vi "create_or_update_indexFile.vi"(1 "html code":string, 2 "folder name":string) -> (0 "status":string)   [LabVIEW 2014]
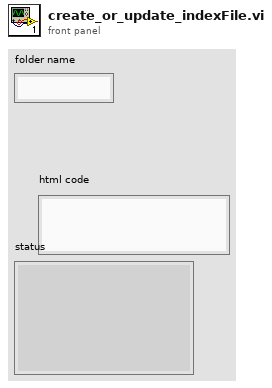
[diagram p1: front panel]
types:
  T1 = enum16{"open", "replace", "create", "open or create", "replace or create", "replace or create with confirmation"}
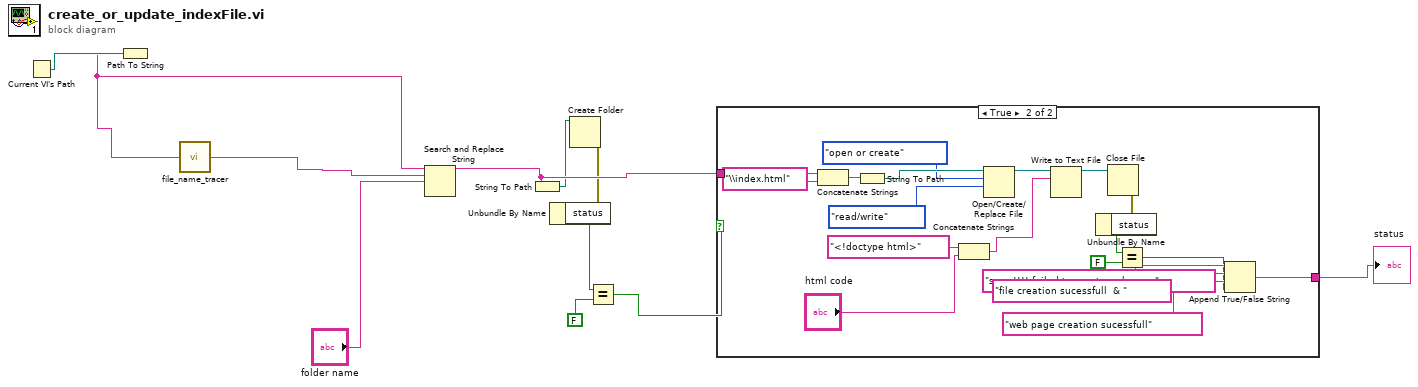
[diagram p0: block diagram]
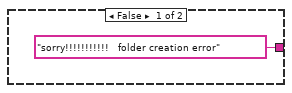
[diagram p2: hidden frame]
diagram:
  n1 = Current VI's Path() -> (path=w8:path)
  n2 = Path To String(path=w8) -> (string=w2:string)
  n3 = call "file_name_tracer.vi"("input path string"=w2) -> ("file name"=w1:string)
  n4 = Search and Replace String(input string=w2, search string=w1, replace string="folder name") -> (result string=w9:string)  [unwired: 5 in, 3 out]
  n5 = String To Path(string=w9) -> (path=w7:path)
  n6 = Create Folder(path (use dialog)=w7) -> (error out=w6:errorcluster)  [unwired: 2 in, 2 out]
  n7 = Unbundle By Name(w6) -> ("status"=w5:bool)
  n8 = Equal?(x=w5, y=FALSE) -> (x = y?=w11:bool)
  n9 = case shown="True" w11 {
    tunnel: ["sorry!!!!!!!!!!!   folder creation error" ("output string") w14] -> w10
    tunnel: w9 -> [_ w13]
    frame False {
    }
    frame True {
      n10 = Concatenate Strings(w13, "\\index.html" ("string")) -> (w30:string)
      n11 = String To Path(string=w30) -> (path=w29:path)
      n12 = Concatenate Strings("<!doctype html>" ("string"), "html code") -> (w23:string)
      n13 = Open/Create/Replace File(file path (use dialog)=w29, operation (0:open)=T1."open or create", access (0:read/write)=enum16{"read/write", "read-only", "write-only"}."read/write") -> (refnum out=w26:refnum<file>)  [unwired: 3 in, 2 out]
      n14 = Write to Text File(file (use dialog)=w26, text=w23) -> (refnum out=w22:refnum<file>)  [unwired: 2 in, 2 out]
      n15 = Close File(refnum=w22) -> (error out=w21:errorcluster)  [unwired: 1 in, 1 out]
      n16 = Unbundle By Name(w21) -> ("status"=w20:bool)
      n17 = Equal?(x=w20, y=FALSE) -> (x = y?=w15:bool)
      n18 = Append True/False String(1:w15, 2:"sorry!!!! failed to create web page" ("false string"), 3:"web page creation sucessfull" ("true string"), 4:"file creation sucessfull  & " ("string (\"\")")) -> (0:w14:string)
    }
  }
  "status" <- w10
